vi "9_2.vi"() -> ()   [LabVIEW 2021, in "2022.lvlib"]
uses:
  2022.lvlib
  <vilib>/Analysis/Matrix/NI_Matrix.lvlib
  <vilib>/Analysis/Matrix/Numeric/Conversions/Array To Matrix - RA2.vi
  <userlib>/_OpenG.lib/array/array.llb/Remove Duplicates from 1D Array (Variant)__ogtk.vi
panel:
  out "size(s)":i32
  out "data":cluster{"PosX":i32, "PosY":i32}[](array[cluster])
  out "Output Array":variant[](array[variant])
  out "Array":cluster{"PosX":i32, "PosY":i32}[](array[cluster])
  out "output cluster":cluster{"PosX":i32, "PosY":i32}
  out "subarray":string[](array[string])
  out "initialized array":dbl[][](array[numeric])
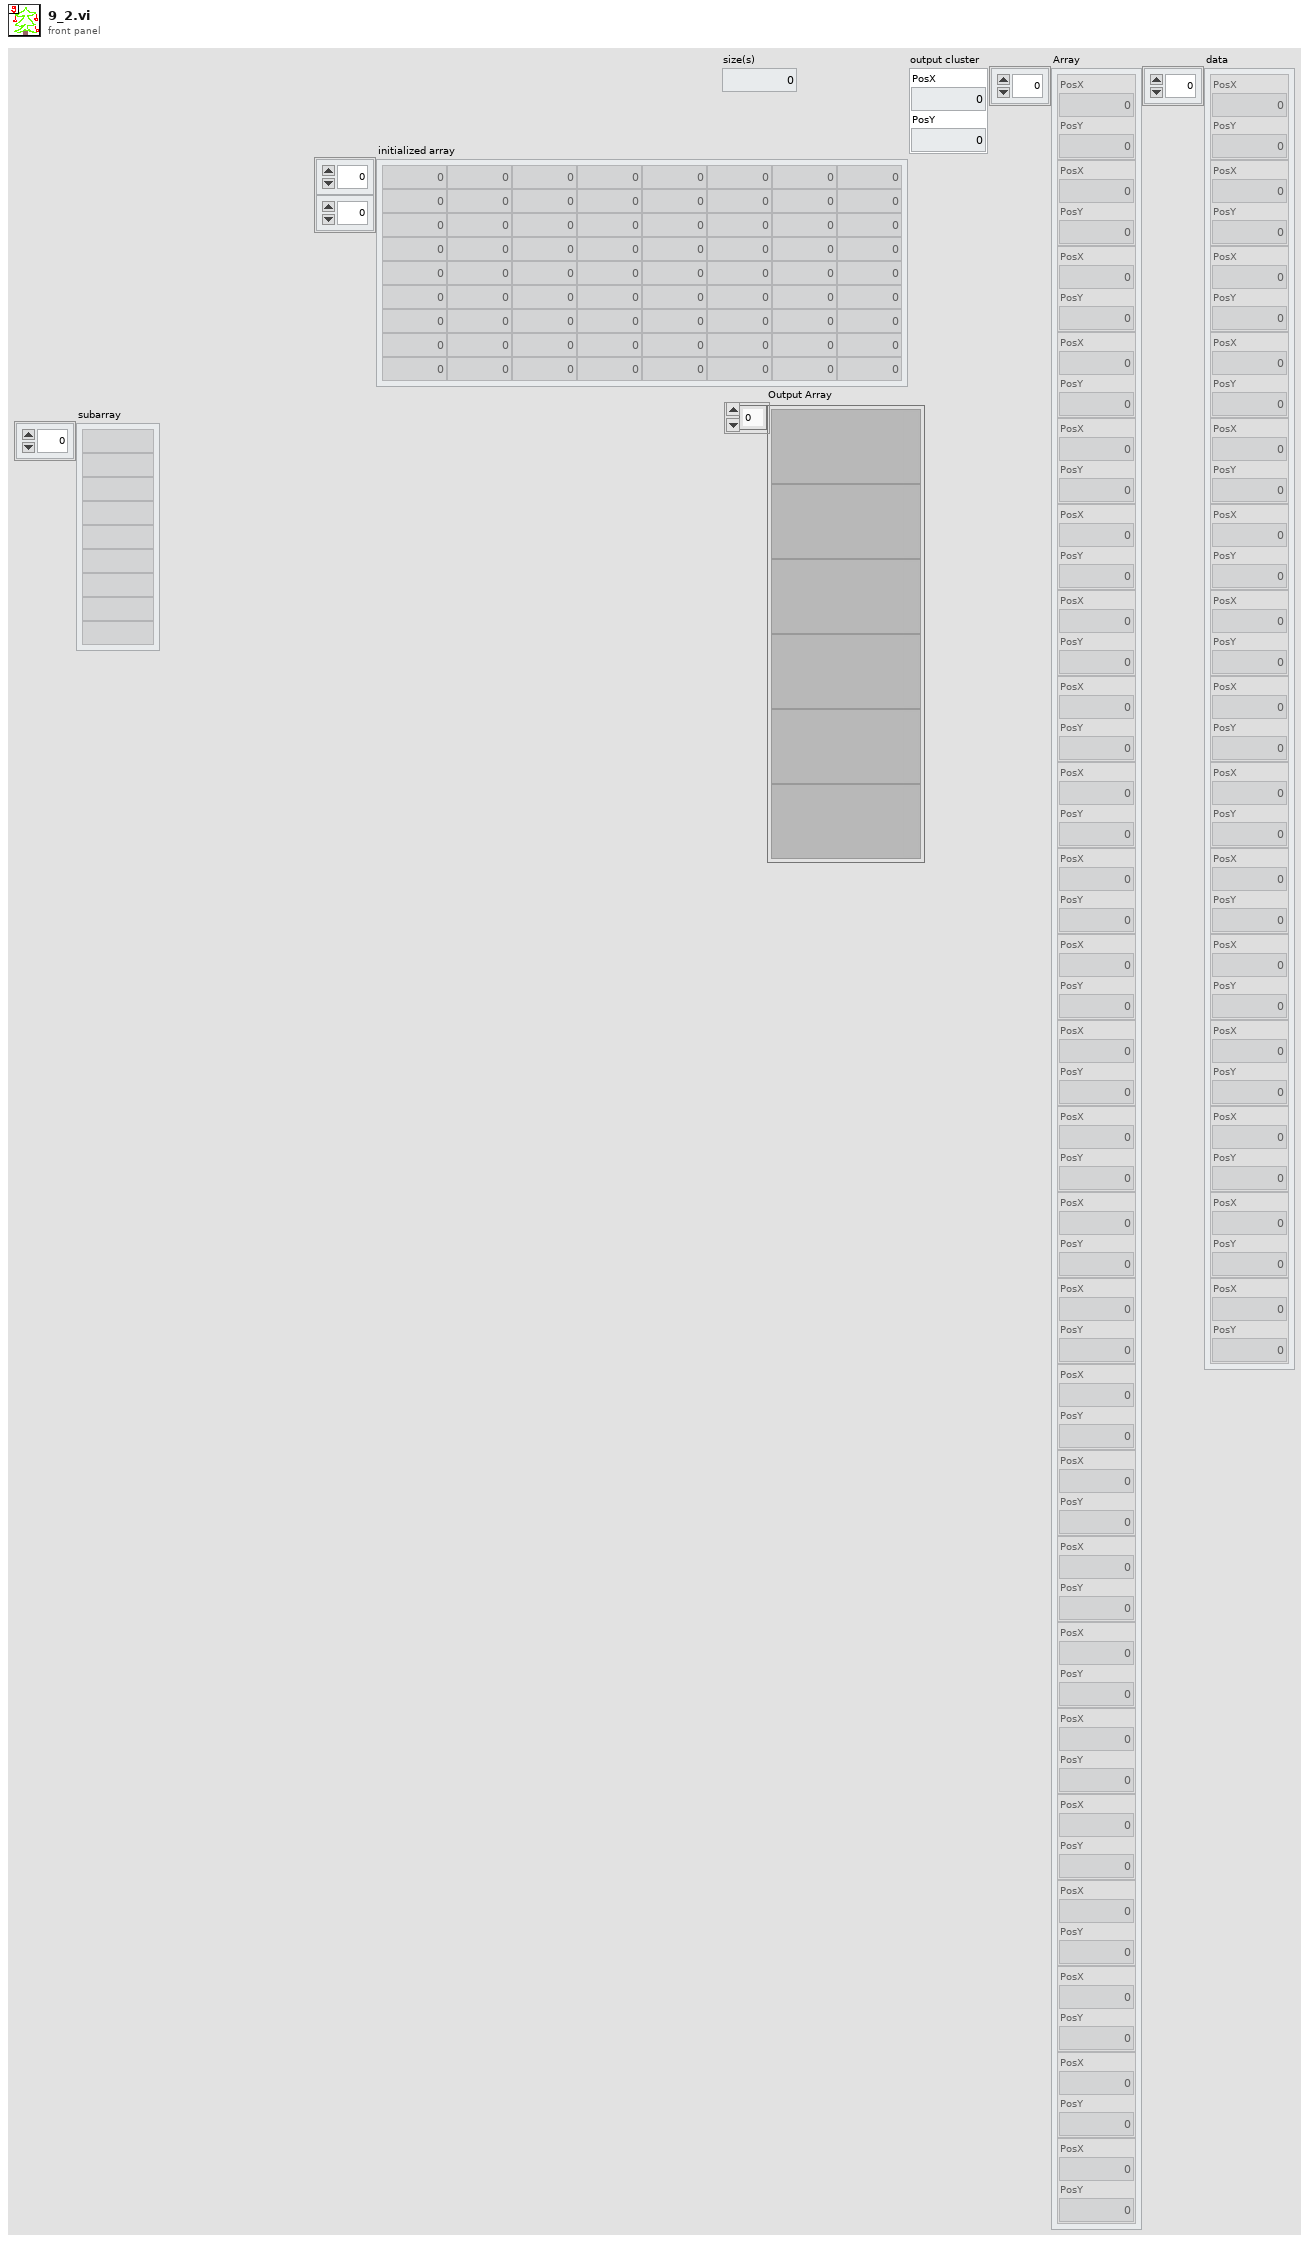
[diagram p1: front panel]
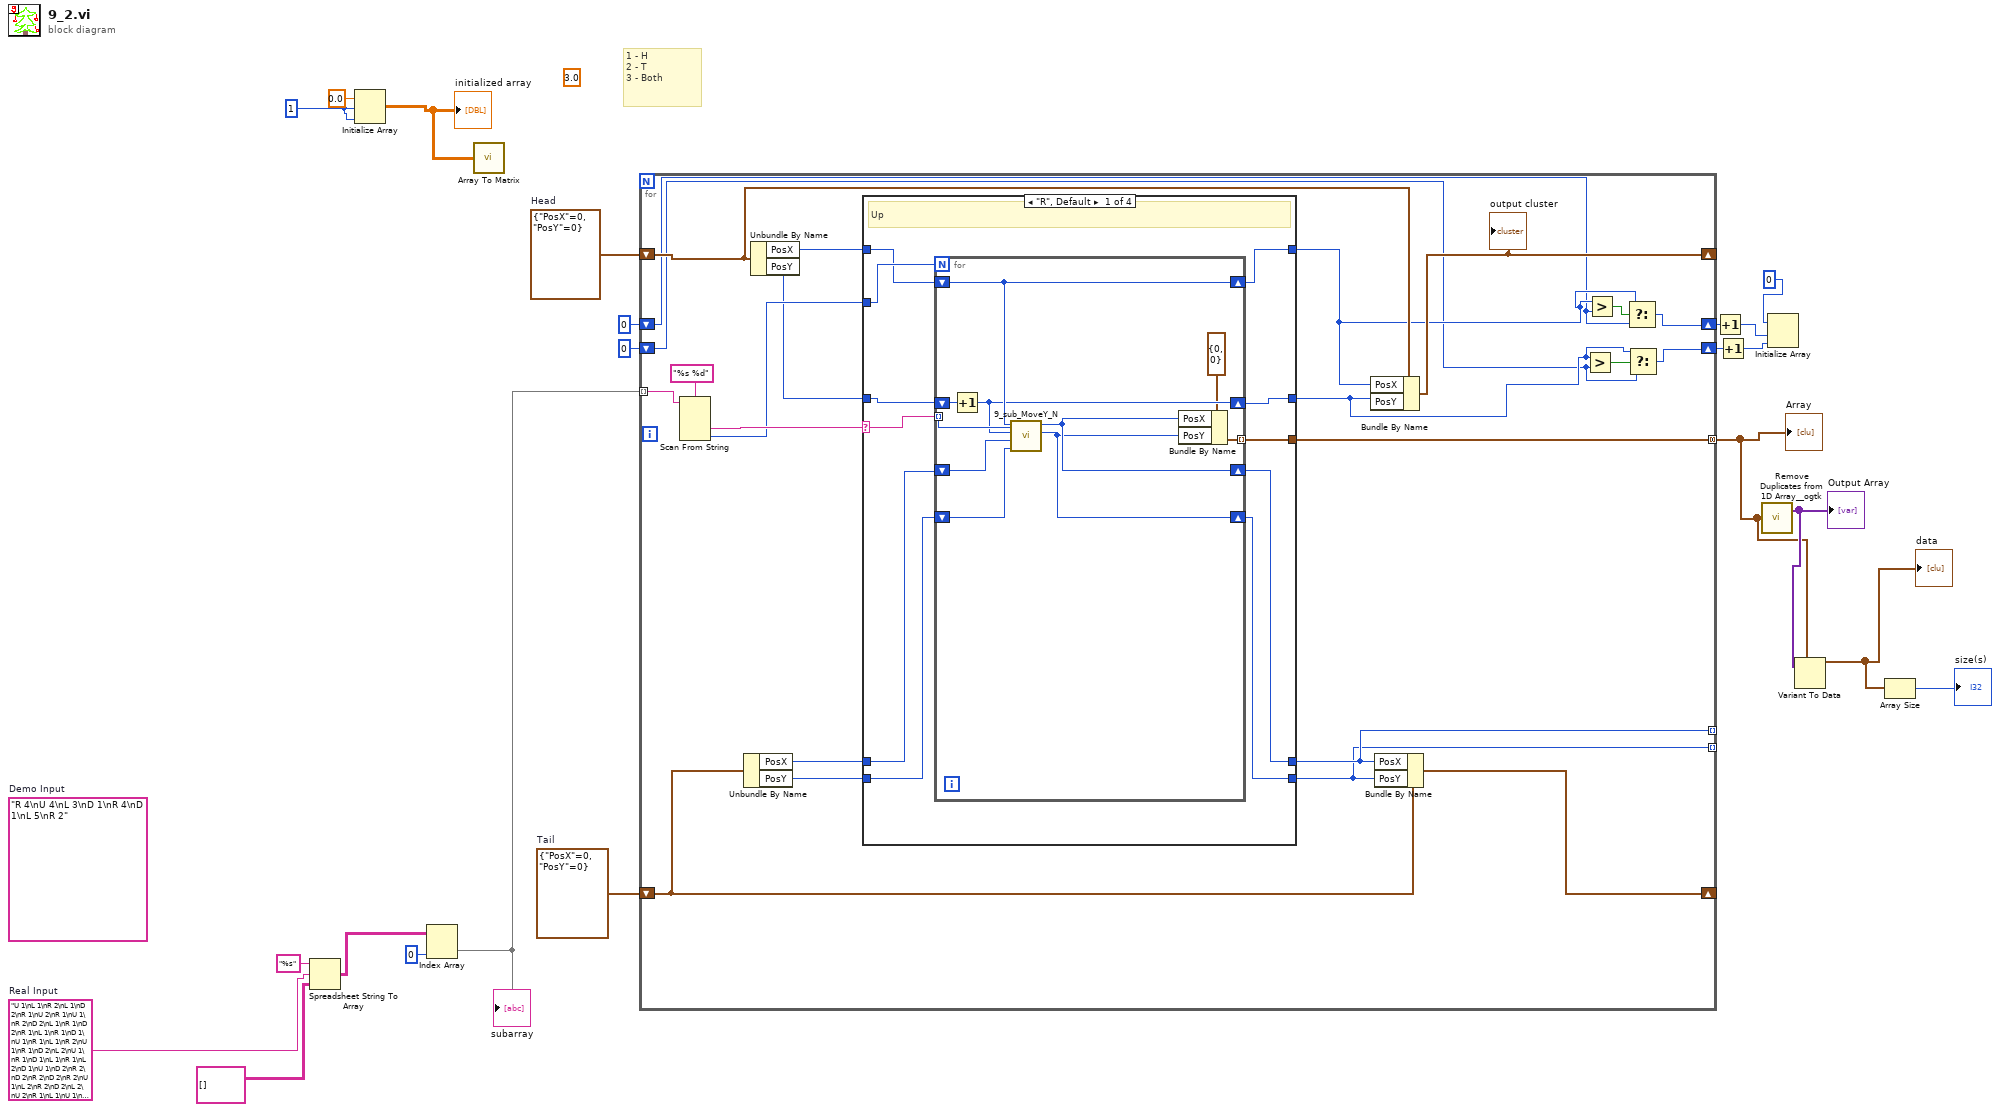
[diagram p0: block diagram]
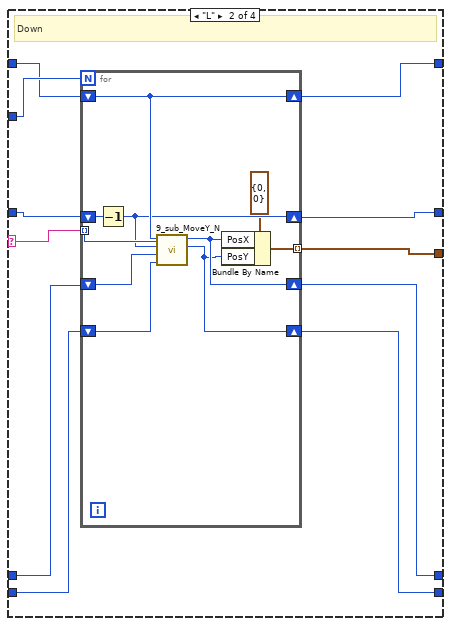
[diagram p2: hidden frame]
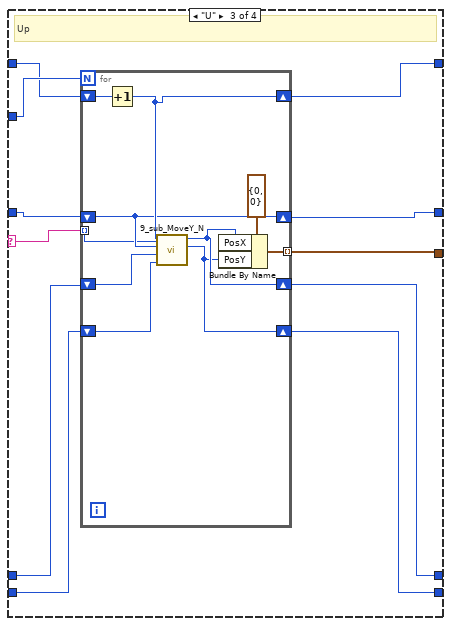
[diagram p3: hidden frame]
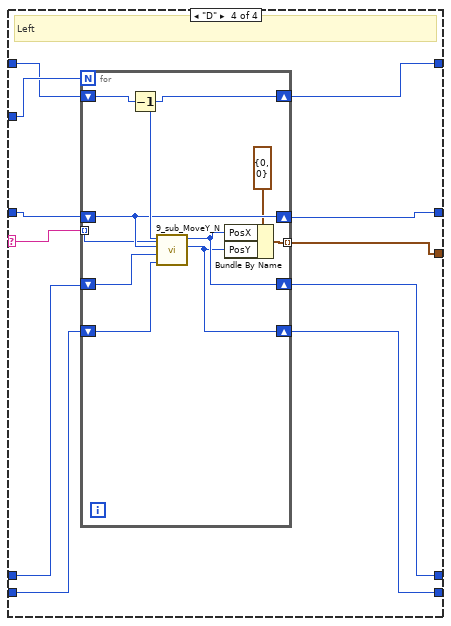
[diagram p4: hidden frame]
diagram:
  w13 = cluster{"PosX":i32, "PosY":i32} {"PosX"=0, "PosY"=0}  # Tail
  w14 = cluster{"PosX":i32, "PosY":i32} {"PosX"=0, "PosY"=0}  # Head
  (unwired) 3.0 ("new element/submatrix")
  w21 = 1 ("dimension size")
  (unwired) "R 4\nU 4\nL 3\nD 1\nR 4\nD 1\nL 5\nR 2"  # Demo Input
  w1 = "U 1\nL 1\nR 2\nL 1\nD 2\nR 1\nU 2\nR 1\nU 1\nR 2\nD 2\nL 1\nR 1\nD 2\nR 1\nL 1\nR 1\nD 1\nU 1\nR 1\nL 1\nR 2\nU 1\nR 1\nD 2\nL 2\nU 1\nR 1\nD 1\nL 1\nR 1\nL 2\nD 1\nU 1\nD 2\nR 2\nD 2\nR 2\nD 2\nR 2\nU 1\nL 2\nR 2\nD 2\nL 2\nU 2\nR 1\nL 1\nU 1\nR 1\nD 1\nR 1\nL 1\nR 1\nD 2\nL 2\nU 1\nR 1\nL 1\nR 1\nU 2\nD 2\nU 2\nL 1\nU 2\nL 1\nR 2\nU 2\nD 1\nL 1\nR 1\nL 2\nU 1\nD 2\nR 2\nU 2\nR 1\nL 1\nU 2\nR 2\nL 1\nR 2\nD 1\nU 2\nD 2\nR 2\nL 1\nR 1\nU 2\nD 2\nU 2\nD 1\nU 1\nR 2\nD 1\nR 1\nL 1\nD 2\nL 2\nU 2\nR 2\nU 1\nR 2\nU 1\nD 1\nR 2\nU 1\nR 1\nU 2\nR 2\nD 2\nL 2\nD 3\nR 2\nU 2\nR 2\nU 2\nL 3\nU 1\nL 1\nR 3\nD 2\nR 2\nU 1\nL 2\nD 2\nL 3\nU 3\nD 2\nR 3\nU 3\nR 2\nD 2\nU 3\nL 1\nU 2\nR 2\nL 1\nD 3\nU 1\nR 3\nL 2\nD 1\nU 2\nL 3\nR 3\nU 3\nL 1\nD 1\nR 3\nD 3\nR 1\nU 2\nR 3\nL 2\nR 1\nU 2\nL 3\nD 1\nR 3\nU 2\nD 2\nR 2\nD 3\nL 3\nD 1\nL 2\nD 1\nR 2\nL 1\nD 2\nU 1\nD 3\nU 1\nR 1\nU 1\nR 3\nL 3\nU 2\nD 3\nR 3\nU 1\nL 1\nR 1\nU 3\nL 2\nU 2\nD 3\nL 2\nD 1\nR 2\nD 2\nL 1\nR 2\nU 1\nD 3\nR 3\nD 2\nR 3\nL 3\nR 3\nD 1\nU 1\nR 1\nU 2\nD 2\nL 2\nD 3\nR 2\nD 3\nU 2\nL 2\nR 1\nU 3\nL 1\nD 1\nU 1\nD 2\nU 1\nL 3\nR 2\nD 1\nL 3\nU 1\nR 3\nD 2\nU 4\nD 1\nL 4\nR 2\nL 2\nR 2\nU 4\nR 1\nU 3\nL 2\nU 2\nR 3\nL 3\nD 3\nR 4\nD 4\nR 3\nD 1\nL 4\nD 4\nU 3\nD 3\nL 4\nR 4\nL 2\nR 3\nL 4\nD 3\nL 3\nU 1\nR 2\nU 1\nL 3\nU 4\nD 1\nL 2\nU 2\nL 1\nD 1\nR 2\nL 4\nR 3\nU 4\nR 1\nD 1\nR 1\nU 3\nD 4\nR 1\nU 4\nR 2\nD 2\nU 2\nR 2\nU 4\nL 1\nD 3\nL 4\nD 2\nL 2\nD 2\nU 4\nL 4\nR 1\nD 1\nR 3\nD 3\nL 4\nR 3\nD 2\nR 1\nD 1\nR 1\nU 1\nD 1\nL 1\nD 1\nR 2\nL 3\nD 1\nR 1\nL 4\nD 4\nR 4\nL 3\nD 4\nU 2\nL 1\nD 3\nU 2\nD 1\nR 2\nD 2\nL 2\nU 1\nD 4\nR 3\nU 4\nD 1\nR 3\nU 1\nD 1\nU 1\nR 1\nD 1\nR 3\nU 4\nR 4\nU 2\nL 1\nU 1\nL 3\nR 5\nD 2\nU 1\nR 3\nD 3\nR 1\nD 1\nL 5\nR 1\nD 1\nR 2\nU 3\nR 2\nL 4\nU 3\nD 4\nU 1\nR 3\nD 1\nR 2\nL 3\nR 3\nU 2\nL 5\nU 3\nR 4\nD 4\nR 2\nD 3\nR 2\nU 4\nL 5\nR 2\nL 3\nU 4\nL 5\nR 3\nD 3\nU 4\nR 2\nU 5\nR 2\nU 5\nD 1\nL 2\nD 2\nU 3\nR 3\nL 3\nU 3\nD 5\nR 4\nD 4\nL 4\nD 5\nR 1\nU 4\nL 2\nR 1\nD 3\nL 2\nR 2\nL 3\nR 2\nL 2\nD 3\nU 5\nD 5\nL 3\nR 5\nU 3\nL 3\nD 5\nL 4\nD 1\nL 2\nD 4\nU 4\nD 1\nR 1\nL 4\nR 3\nU 2\nL 3\nU 4\nD 4\nR 2\nD 4\nU 2\nD 4\nU 2\nL 4\nD 5\nL 4\nR 1\nL 2\nR 3\nD 2\nR 5\nL 1\nU 5\nR 1\nD 5\nL 1\nD 2\nU 5\nD 2\nU 1\nD 6\nU 2\nL 5\nD 2\nR 1\nD 1\nR 1\nD 5\nU 1\nD 5\nR 4\nL 3\nR 4\nU 1\nD 5\nU 5\nL 4\nU 5\nL 4\nU 5\nR 2\nL 6\nD 4\nL 1\nU 1\nR 6\nD 4\nL 1\nD 2\nR 2\nU 5\nR 5\nU 4\nL 5\nR 4\nD 4\nU 4\nD 1\nR 2\nL 5\nU 3\nR 1\nL 3\nU 6\nR 5\nL 2\nD 4\nR 4\nU 5\nR 2\nU 6\nL 4\nU 6\nR 2\nL 6\nD 5\nR 6\nU 1\nL 3\nU 4\nR 2\nL 5\nD 4\nL 6\nU 1\nD 1\nR 2\nD 5\nL 1\nR 5\nL 3\nU 5\nD 4\nU 5\nD 4\nU 2\nR 4\nL 3\nD 4\nL 5\nR 6\nU 6\nD 5\nU 2\nR 4\nD 5\nL 5\nR 3\nL 3\nD 3\nU 6\nL 1\nD 3\nR 2\nL 3\nR 2\nL 6\nD 1\nL 6\nD 4\nL 6\nR 4\nD 5\nL 3\nU 6\nR 5\nU 4\nD 1\nL 5\nU 1\nD 2\nU 2\nD 5\nR 7\nL 3\nU 5\nR 4\nL 5\nU 1\nR 2\nD 6\nL 6\nD 2\nL 1\nD 6\nU 2\nD 2\nU 2\nD 6\nL 1\nR 6\nU 7\nD 2\nL 3\nR 3\nU 6\nD 3\nR 4\nU 3\nL 7\nD 3\nU 6\nD 2\nU 1\nR 4\nL 1\nR 3\nU 5\nD 6\nR 2\nL 4\nD 5\nR 6\nL 5\nD 1\nR 3\nD 2\nL 7\nU 1\nR 5\nD 6\nU 6\nD 4\nU 6\nD 2\nL 2\nU 7\nD 1\nR 3\nU 3\nR 1\nL 6\nD 7\nL 4\nR 1\nD 7\nL 2\nU 6\nD 2\nR 6\nD 7\nU 7\nR 5\nL 1\nU 3\nR 5\nD 4\nU 2\nD 2\nL 6\nD 2\nU 7\nR 4\nL 7\nU 4\nD 6\nU 2\nD 6\nL 3\nU 5\nR 5\nD 4\nR 1\nD 6\nU 6\nR 3\nL 2\nU 1\nR 7\nD 4\nL 2\nD 4\nL 5\nU 3\nR 6\nL 3\nD 7\nR 7\nL 1\nU 4\nL 6\nR 7\nU 3\nR 1\nD 8\nL 3\nD 3\nU 3\nR 2\nL 6\nU 4\nL 2\nD 7\nL 5\nD 1\nR 3\nU 2\nL 6\nR 2\nU 1\nD 6\nU 4\nD 1\nU 8\nD 7\nR 3\nL 3\nR 1\nD 1\nR 5\nL 5\nR 6\nU 4\nR 4\nU 3\nR 4\nL 6\nR 4\nU 6\nL 5\nU 8\nL 1\nD 1\nL 4\nU 8\nR 2\nU 7\nL 4\nU 7\nL 7\nD 5\nU 1\nR 7\nU 7\nD 6\nR 5\nU 5\nD 2\nR 8\nL 1\nD 3\nL 5\nD 5\nR 1\nU 1\nR 4\nD 3\nR 1\nU 4\nR 8\nD 3\nL 4\nR 7\nL 4\nR 7\nL 7\nR 1\nL 1\nD 2\nL 6\nR 7\nD 5\nU 7\nL 8\nU 1\nL 8\nU 2\nR 6\nL 4\nU 1\nR 1\nU 3\nL 6\nD 7\nL 3\nD 2\nR 4\nU 5\nD 1\nU 2\nD 6\nL 6\nU 4\nD 1\nL 2\nR 4\nU 2\nL 1\nR 5\nL 3\nR 5\nU 7\nR 4\nL 4\nR 2\nD 4\nL 1\nR 2\nD 1\nL 2\nR 2\nU 2\nR 5\nL 7\nU 3\nR 1\nD 5\nU 7\nD 8\nR 7\nD 5\nU 2\nL 5\nD 4\nL 2\nD 8\nU 7\nD 3\nU 4\nL 9\nD 2\nU 7\nR 7\nD 9\nU 3\nR 2\nL 7\nU 5\nL 9\nD 5\nR 6\nD 5\nR 1\nD 1\nR 5\nD 3\nU 2\nR 5\nD 8\nU 4\nR 9\nU 5\nL 2\nU 2\nR 5\nD 9\nU 2\nD 3\nR 4\nD 5\nU 7\nL 2\nU 8\nR 7\nL 1\nU 4\nD 6\nR 8\nU 3\nD 4\nU 1\nR 5\nU 8\nD 9\nU 5\nD 9\nR 7\nD 3\nL 1\nD 4\nR 8\nD 8\nU 5\nD 7\nL 5\nU 1\nD 6\nL 7\nD 1\nR 1\nU 2\nL 3\nR 4\nL 1\nD 7\nL 3\nU 9\nR 1\nU 9\nL 7\nR 1\nU 5\nL 4\nU 8\nD 9\nU 3\nD 9\nR 5\nU 8\nL 9\nU 9\nD 7\nR 7\nL 2\nU 9\nR 7\nU 10\nD 7\nL 1\nD 2\nR 4\nD 9\nL 4\nD 7\nR 9\nU 1\nD 4\nU 8\nL 9\nR 9\nD 3\nR 2\nD 7\nU 2\nD 7\nU 1\nR 3\nD 1\nU 10\nD 5\nU 6\nD 1\nR 5\nD 6\nU 1\nR 6\nU 2\nD 5\nU 8\nL 9\nD 1\nU 9\nD 6\nL 10\nR 4\nD 1\nL 6\nR 1\nL 3\nD 4\nR 9\nD 7\nR 4\nD 8\nR 8\nL 5\nU 7\nR 3\nU 5\nD 4\nL 5\nD 7\nL 10\nU 3\nD 9\nR 7\nU 4\nD 3\nR 7\nU 5\nD 10\nR 1\nL 7\nU 7\nR 5\nU 4\nL 7\nD 6\nR 1\nD 1\nR 4\nL 3\nR 4\nD 3\nL 7\nD 7\nL 6\nR 4\nL 1\nD 2\nU 4\nD 8\nL 8\nR 1\nU 4\nD 1\nU 2\nL 1\nR 4\nU 7\nD 9\nU 4\nD 10\nU 5\nR 3\nD 6\nU 7\nD 6\nL 7\nR 7\nL 7\nR 6\nD 4\nU 4\nL 7\nU 9\nL 6\nD 2\nL 2\nU 10\nL 4\nU 3\nD 3\nL 5\nU 10\nD 10\nR 8\nD 2\nL 6\nD 9\nR 7\nL 8\nR 3\nU 1\nD 4\nU 2\nR 4\nU 5\nD 8\nU 6\nL 4\nU 9\nR 5\nU 8\nL 11\nD 11\nU 6\nD 4\nU 3\nR 7\nL 8\nR 5\nD 5\nU 5\nR 1\nU 10\nL 4\nD 6\nU 11\nR 3\nD 10\nU 10\nL 7\nR 11\nU 9\nL 10\nU 10\nL 11\nD 2\nL 9\nD 3\nL 11\nD 2\nU 1\nD 5\nL 6\nU 3\nD 10\nR 8\nU 10\nR 9\nL 1\nD 6\nU 6\nD 6\nL 8\nR 3\nU 1\nD 2\nL 6\nR 10\nU 7\nD 2\nL 5\nD 10\nU 5\nD 9\nR 4\nL 9\nD 6\nU 9\nR 5\nL 9\nU 1\nD 2\nR 2\nL 5\nR 4\nD 8\nU 8\nD 11\nL 4\nD 3\nU 1\nL 9\nR 8\nL 10\nR 8\nL 10\nU 10\nD 5\nR 11\nU 2\nR 8\nU 1\nL 6\nU 5\nD 2\nU 2\nR 3\nL 4\nR 1\nD 6\nL 6\nU 5\nR 1\nL 6\nD 1\nR 5\nL 2\nR 11\nD 5\nL 6\nR 1\nD 11\nU 9\nD 12\nU 8\nR 7\nL 6\nR 9\nU 7\nD 2\nR 5\nD 12\nL 10\nD 7\nL 5\nU 7\nD 9\nR 7\nU 8\nD 3\nU 8\nD 5\nU 1\nL 10\nU 7\nL 2\nR 5\nL 2\nU 1\nL 8\nR 2\nD 8\nR 9\nD 9\nR 11\nD 4\nR 3\nU 2\nD 9\nR 12\nU 11\nD 8\nR 6\nD 9\nU 3\nL 5\nR 1\nU 4\nR 4\nU 10\nR 11\nU 5\nR 9\nU 1\nR 5\nD 3\nR 8\nU 3\nR 6\nU 4\nR 3\nD 2\nL 2\nU 7\nL 2\nU 12\nD 10\nL 7\nU 6\nR 7\nU 1\nL 11\nU 12\nR 12\nL 12\nD 10\nR 9\nU 12\nL 6\nU 2\nL 7\nU 11\nR 7\nU 6\nL 3\nU 3\nD 1\nU 11\nR 1\nD 4\nR 10\nL 10\nR 6\nD 11\nR 1\nD 5\nL 1\nR 1\nL 4\nR 7\nU 12\nR 6\nL 10\nD 12\nL 4\nR 8\nU 5\nL 7\nR 10\nD 13\nU 7\nD 1\nR 1\nD 9\nR 3\nD 1\nL 4\nD 3\nR 5\nU 9\nR 11\nL 4\nR 1\nD 11\nL 2\nR 4\nD 7\nR 3\nU 2\nD 6\nR 2\nL 13\nR 5\nL 4\nR 4\nU 13\nR 3\nU 4\nR 3\nD 1\nL 3\nU 6\nL 8\nU 5\nR 4\nD 10\nL 3\nU 10\nR 11\nD 11\nU 2\nD 2\nR 4\nU 2\nD 1\nR 10\nU 5\nL 9\nU 11\nR 10\nD 4\nL 1\nU 5\nR 4\nU 6\nR 9\nD 12\nL 10\nR 5\nL 5\nD 9\nU 2\nR 7\nU 2\nR 5\nL 8\nD 5\nR 1\nD 5\nR 8\nU 11\nR 7\nL 13\nU 10\nD 3\nU 1\nD 2\nL 1\nD 12\nL 9\nD 12\nR 5\nU 8\nR 6\nL 6\nR 5\nU 7\nL 10\nD 5\nU 11\nD 4\nU 8\nR 7\nU 8\nR 2\nL 10\nD 5\nL 10\nD 3\nU 13\nD 11\nU 3\nR 10\nU 9\nD 7\nU 6\nR 1\nU 9\nR 11\nD 7\nR 6\nU 9\nR 6\nU 12\nD 6\nR 13\nL 14\nU 10\nR 9\nL 13\nR 7\nD 9\nU 12\nL 8\nD 5\nR 3\nU 5\nR 10\nL 4\nD 5\nR 4\nD 2\nL 12\nR 8\nD 9\nR 5\nD 7\nU 5\nD 11\nL 13\nD 12\nR 2\nU 5\nL 1\nU 2\nL 6\nU 9\nD 10\nL 3\nD 8\nR 12\nU 9\nR 9\nU 9\nR 8\nU 6\nL 10\nU 5\nR 9\nD 2\nU 12\nD 3\nR 12\nL 10\nD 5\nL 7\nD 9\nL 5\nR 7\nD 8\nU 10\nL 11\nR 9\nL 13\nR 8\nU 9\nD 8\nU 9\nR 10\nL 4\nU 1\nD 10\nL 1\nD 4\nL 1\nU 13\nR 8\nL 3\nD 5\nR 5\nU 4\nR 5\nU 6\nL 14\nR 5\nU 8\nL 7\nD 7\nR 4\nU 4\nL 14\nU 7\nR 14\nD 3\nU 10\nL 7\nR 5\nL 5\nR 15\nL 3\nD 15\nL 6\nR 3\nL 10\nU 7\nL 2\nR 7\nL 1\nR 8\nU 12\nD 6\nU 11\nD 12\nU 9\nR 2\nD 14\nL 4\nU 9\nD 15\nR 8\nD 9\nL 9\nD 14\nU 5\nR 14\nD 15\nR 6\nL 3\nU 13\nR 13\nU 5\nD 14\nL 2\nD 12\nU 6\nR 5\nU 5\nL 6\nR 5\nD 12\nU 9\nL 7\nD 15\nR 5\nU 7\nD 1\nR 2\nL 11\nU 8\nR 3\nD 3\nU 6\nD 15\nU 2\nD 11\nR 6\nU 9\nD 7\nU 3\nL 13\nU 3\nL 15\nR 10\nL 6\nD 15\nL 3\nU 5\nR 13\nD 13\nL 5\nR 8\nD 2\nR 8\nL 9\nR 7\nL 5\nU 3\nD 11\nR 13\nU 15\nD 5\nR 4\nU 11\nR 14\nL 1\nU 6\nL 13\nR 14\nL 12\nD 5\nR 3\nD 4\nR 5\nU 8\nR 11\nD 8\nU 5\nR 9\nD 8\nR 4\nU 5\nL 7\nD 6\nU 4\nL 2\nD 15\nU 5\nR 16\nL 4\nR 1\nD 12\nL 2\nR 6\nD 6\nR 14\nU 6\nL 14\nR 12\nD 8\nR 1\nU 2\nR 3\nD 7\nR 4\nL 2\nU 6\nL 1\nU 7\nL 12\nR 11\nD 13\nU 16\nR 15\nD 14\nU 13\nD 15\nR 11\nU 12\nR 5\nD 8\nR 2\nL 14\nR 10\nL 16\nU 10\nD 13\nL 11\nU 10\nR 5\nD 7\nL 15\nD 12\nL 4\nR 16\nU 8\nR 8\nL 7\nU 9\nR 7\nU 16\nR 2\nU 5\nR 5\nD 4\nL 7\nD 5\nL 4\nU 13\nD 9\nR 2\nD 2\nU 5\nL 3\nD 16\nR 13\nL 10\nR 7\nL 9\nR 3\nL 5\nD 10\nL 10\nR 2\nL 13\nR 5\nL 11\nR 16\nU 12\nR 11\nD 12\nR 7\nL 2\nU 12\nD 11\nU 12\nL 1\nR 6\nU 3\nL 3\nD 1\nR 5\nU 6\nL 15\nR 8\nD 5\nL 16\nD 13\nR 15\nD 14\nR 4\nU 15\nR 5\nL 8\nD 12\nU 11\nD 13\nL 9\nD 13\nL 7\nU 9\nR 15\nU 13\nD 16\nR 6\nL 8\nR 7\nU 4\nR 10\nU 7\nD 10\nU 8\nD 7\nL 17\nR 7\nL 8\nD 5\nL 5\nU 15\nD 6\nL 1\nD 2\nR 17\nL 6\nD 15\nR 4\nL 2\nR 10\nD 4\nR 6\nD 11\nU 1\nL 17\nD 11\nU 6\nD 17\nR 15\nL 13\nD 9\nR 12\nU 13\nR 2\nL 12\nD 1\nR 17\nU 13\nD 15\nU 7\nR 8\nD 6\nR 8\nD 16\nU 16\nD 2\nU 1\nR 7\nU 15\nL 7\nR 12\nU 10\nD 4\nR 17\nD 11\nR 12\nD 8\nL 3\nR 3\nD 5\nR 17\nL 15\nU 11\nR 1\nL 4\nR 6\nD 6\nU 2\nL 1\nD 2\nU 1\nD 11\nL 1\nR 11\nD 7\nU 16\nL 14\nU 5\nR 13\nD 9\nU 17\nD 3\nR 12\nU 16\nR 10\nL 17\nD 5\nU 16\nD 12\nL 2\nR 16\nL 17\nU 4\nR 15\nD 4\nL 11\nU 3\nR 17\nD 8\nR 7\nD 15\nR 14\nD 6\nR 5\nL 1\nD 5\nL 11\nD 5\nU 13\nL 13\nU 8\nD 8\nL 13\nD 1\nL 10\nU 14\nR 7\nL 11\nD 4\nR 16\nD 3\nL 9\nR 3\nD 4\nL 4\nU 2\nR 13\nD 18\nU 15\nD 7\nL 18\nU 3\nD 17\nU 13\nR 9\nL 8\nR 9\nU 16\nR 14\nD 17\nL 16\nR 3\nU 4\nD 1\nR 8\nD 14\nL 14\nU 17\nL 16\nR 15\nD 9\nU 13\nR 14\nU 9\nD 13\nR 2\nL 3\nD 8\nU 5\nR 1\nL 5\nR 4\nU 8\nL 7\nU 5\nR 11\nD 17\nL 4\nU 3\nR 1\nU 18\nD 1\nU 6\nR 2\nD 16\nU 15\nD 8\nL 13\nR 2\nU 16\nL 9\nD 1\nU 9\nR 5\nL 16\nD 2\nL 2\nR 8\nD 17\nR 13\nU 5\nR 6\nU 2\nL 12\nR 2\nD 14\nR 14\nL 11\nR 1\nL 9\nD 18\nL 4\nU 4\nD 15\nL 14\nR 15\nU 6\nD 3\nR 15\nL 12\nU 3\nD 12\nU 13\nL 6\nU 17\nD 6\nL 10\nR 16\nL 7\nU 2\nD 1\nR 10\nU 11\nR 1\nU 19\nD 5\nL 11\nD 14\nL 17\nU 16\nL 13\nR 4\nL 16\nD 10\nL 4\nD 9\nR 19\nL 19\nR 12\nL 12\nD 8\nL 6\nD 14\nU 7\nD 13\nU 18\nD 13\nU 6\nD 6\nR 18\nU 18\nD 15\nL 14\nR 7\nD 11\nR 4\nL 14\nR 5\nD 4\nL 12\nD 16\nR 17\nU 15\nL 9\nU 10\nR 7\nD 10\nL 3\nU 15\nL 1\nD 15\nU 1\nD 12\nL 4\nD 10\nU 6\nR 6\nL 11\nD 5\nR 1\nD 11\nU 16\nL 16\nR 19\nU 8\nR 11\nD 17\nL 19\nR 6\nU 7\nR 2\nD 9\nR 11\nD 17\nU 17\nD 4\nR 8\nD 6\nU 10\nR 3\nL 17\nD 5\nR 19\nU 1\nL 5\nU 5\nD 6\nU 6\nL 18\nR 18\nL 4\nR 12\nD 14\nL 17\nR 8\nL 13\nR 6\nL 14\nD 3\nR 13\nL 16\nD 14\nU 6\nD 6"  # Real Input
  # "1 - H\n2 - T\n3 - Both"
  n1 = Spreadsheet String To Array(format string="%s", spreadsheet string=w1, array type (2D Dbl)=string[][] []) -> (array=w18:string[][])  [unwired: 1 in]
  n2 = Initialize Array(0.0 ("element"), w21, w21) -> (w15:dbl[][])
  "initialized array" <- w15
  n3 = Index Array(array=w18, index (col)=0 ("disabled index (col)")) -> (element=w16:string[])  [unwired: 1 in]
  "subarray" <- w16
  n4 = call-poly <vilib>:"Array To Matrix.vi"("Real 2D Array"=w15) -> ()  [unwired: 1 out]
  n5 = for {
    tunnel: w16 -> [w45] mode=indexing
    shift-right: [w38] -> _
    shift-left: w14 -> [w41]
    shift-right: [w34] -> _
    shift-left: w13 -> [w37]
    shift-right: [w30] -> w9
    shift-left: 0 ("PosX") -> [w31]
    shift-right: [w26] -> w8
    shift-left: 0 ("PosY") -> [w27]
    tunnel: [w25] -> _ mode=indexing
    tunnel: [w24] -> _ mode=indexing
    tunnel: [w23] -> w4 mode=concatenating
    n6 = Scan From String(format string="%s %d", input string=w45) -> (output 1=w43:string, output 2=w42:i32)  [unwired: 4 in, 3 out]
    n7 = Unbundle By Name(w37) -> ("PosX"=w36:i32, "PosY"=w35:i32)
    n8 = Unbundle By Name(w41) -> ("PosX"=w40:i32, "PosY"=w39:i32)
    n9 = case shown="\"R\", Default" w43 {
      selector: w43 -> [w47 w68 w89 w110]
      tunnel: w42 -> [w56 w77 w98 w119]
      tunnel: w40 -> [w55 w76 w97 w118]
      tunnel: w39 -> [w53 w74 w95 w116]
      tunnel: [w54 w75 w96 w117] -> w32
      tunnel: [w52 w73 w94 w115] -> w28
      tunnel: [w49 w70 w91 w112] -> w25
      tunnel: w36 -> [w51 w72 w93 w114]
      tunnel: w35 -> [w50 w71 w92 w113]
      tunnel: [w48 w69 w90 w111] -> w24
      tunnel: [w46 w67 w88 w109] -> w23
      frame "R", Default {
        # "Up"
        n10 = for {
          N: w56 -> [_]
          shift-right: [w66] -> w54
          shift-left: w55 -> [w66]
          shift-right: [w61] -> w52
          shift-left: w53 -> [w65]
          shift-right: [w59] -> w49
          shift-left: w51 -> [w64]
          shift-right: [w58] -> w48
          shift-left: w50 -> [w63]
          tunnel: w47 -> [w62] mode=indexing
          tunnel: [w57] -> w46 mode=indexing
          n11 = Increment(x=w65) -> (x+1=w61:i32)
          n12 = call "9_sub_MoveY_N.vi"("T_y"=w63, "T_x"=w64, "H_y"=w61, "H_x"=w66) -> ("T_y 2"=w58:i32, "T_x 2"=w59:i32, "H_x 2"=w62:i32)  [unwired: 4 in, 1 out]
          n13 = Bundle By Name(cluster=cluster{"PosX":i32, "PosY":i32} {"PosX"=0, "PosY"=0} ("Tail"), "PosX"=w59, "PosY"=w58) -> (w57:cluster{"PosX":i32, "PosY":i32})
        }
      }
      frame "L" {
        # "Down"
        n14 = for {
          N: w77 -> [_]
          shift-right: [w87] -> w75
          shift-left: w76 -> [w87]
          shift-right: [w82] -> w73
          shift-left: w74 -> [w86]
          shift-right: [w80] -> w70
          shift-left: w72 -> [w85]
          shift-right: [w79] -> w69
          shift-left: w71 -> [w84]
          tunnel: w68 -> [w83] mode=indexing
          tunnel: [w78] -> w67 mode=indexing
          n15 = Decrement(x=w86) -> (x-1=w82:i32)
          n16 = call "9_sub_MoveY_N.vi"("T_y"=w84, "T_x"=w85, "H_y"=w82, "H_x"=w87) -> ("T_y 2"=w79:i32, "T_x 2"=w80:i32, "H_x 2"=w83:i32)  [unwired: 4 in, 1 out]
          n17 = Bundle By Name(cluster=cluster{"PosX":i32, "PosY":i32} {"PosX"=0, "PosY"=0} ("Tail"), "PosX"=w80, "PosY"=w79) -> (w78:cluster{"PosX":i32, "PosY":i32})
        }
      }
      frame "U" {
        # "Up"
        n18 = for {
          N: w98 -> [_]
          shift-right: [w107] -> w96
          shift-left: w97 -> [w108]
          shift-right: [w106] -> w94
          shift-left: w95 -> [w106]
          shift-right: [w101] -> w91
          shift-left: w93 -> [w105]
          shift-right: [w100] -> w90
          shift-left: w92 -> [w104]
          tunnel: w89 -> [w103] mode=indexing
          tunnel: [w99] -> w88 mode=indexing
          n19 = Increment(x=w108) -> (x+1=w107:i32)
          n20 = call "9_sub_MoveY_N.vi"("T_y"=w104, "T_x"=w105, "H_y"=w106, "H_x"=w107) -> ("T_y 2"=w100:i32, "T_x 2"=w101:i32, "H_x 2"=w103:i32)  [unwired: 4 in, 1 out]
          n21 = Bundle By Name(cluster=cluster{"PosX":i32, "PosY":i32} {"PosX"=0, "PosY"=0} ("Tail"), "PosX"=w101, "PosY"=w100) -> (w99:cluster{"PosX":i32, "PosY":i32})
        }
      }
      frame "D" {
        # "Left"
        n22 = for {
          N: w119 -> [_]
          shift-right: [w128] -> w117
          shift-left: w118 -> [w129]
          shift-right: [w127] -> w115
          shift-left: w116 -> [w127]
          shift-right: [w122] -> w112
          shift-left: w114 -> [w126]
          shift-right: [w121] -> w111
          shift-left: w113 -> [w125]
          tunnel: w110 -> [w124] mode=indexing
          tunnel: [w120] -> w109 mode=indexing
          n23 = Decrement(x=w129) -> (x-1=w128:i32)
          n24 = call "9_sub_MoveY_N.vi"("T_y"=w125, "T_x"=w126, "H_y"=w127, "H_x"=w128) -> ("T_y 2"=w121:i32, "T_x 2"=w122:i32, "H_x 2"=w124:i32)  [unwired: 4 in, 1 out]
          n25 = Bundle By Name(cluster=cluster{"PosX":i32, "PosY":i32} {"PosX"=0, "PosY"=0} ("Tail"), "PosX"=w122, "PosY"=w121) -> (w120:cluster{"PosX":i32, "PosY":i32})
        }
      }
    }
    n26 = Bundle By Name(cluster=w41, "PosX"=w32, "PosY"=w28) -> (w38:cluster{"PosX":i32, "PosY":i32})
    "output cluster" <- w38
    n27 = Bundle By Name(cluster=w37, "PosX"=w25, "PosY"=w24) -> (w34:cluster{"PosX":i32, "PosY":i32})
    n28 = Greater?(x=w28, y=w27) -> (0:w29:bool)
    n29 = Greater?(x=w32, y=w31) -> (0:w33:bool)
    n30 = Select(t=w32, s=w33, f=w31) -> (s? t:f=w30:i32)
    n31 = Select(t=w28, s=w29, f=w27) -> (s? t:f=w26:i32)
  }
  "Array" <- w4
  n32 = Increment(x=w9) -> (x+1=w7:i32)
  n33 = Increment(x=w8) -> (x+1=w6:i32)
  n34 = call-poly <userlib>:"Remove Duplicates from 1D Array__ogtk.vi"("Input Array"=w4) -> ("Output Array"=w5:variant[])  [unwired: 1 out]
  "Output Array" <- w5
  n35 = Initialize Array(0 ("s? t:f"), w7, w6) -> ()  [unwired: 1 out]
  n36 = Variant To Data(type=w4, Variant=w5) -> (data=w3:cluster{"PosX":i32, "PosY":i32}[])  [unwired: 1 in, 1 out]
  "data" <- w3
  n37 = Array Size(array=w3) -> (size(s)=→"size(s)":i32)
